vi "Write resource name.vi"(8 "error in (no error)":errorcluster, 10 "resource name":string, 11 "_cameraBase in":refnum<class "_cameraBase.lvclass">) -> (0 "error out":errorcluster, 3 "_cameraBase out":refnum<class "_cameraBase.lvclass">)   [LabVIEW 2018, in "_cameraBase.lvclass"]
uses:
  _cameraBase.lvclass
  _cameraBase.lvclass/_cameraBase.ctl
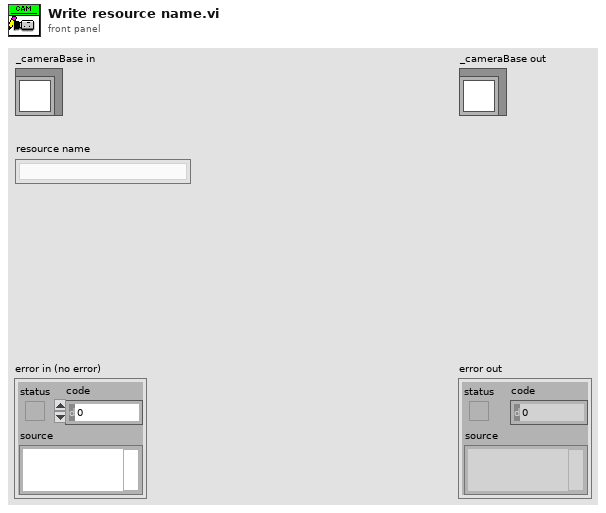
[diagram p1: front panel]
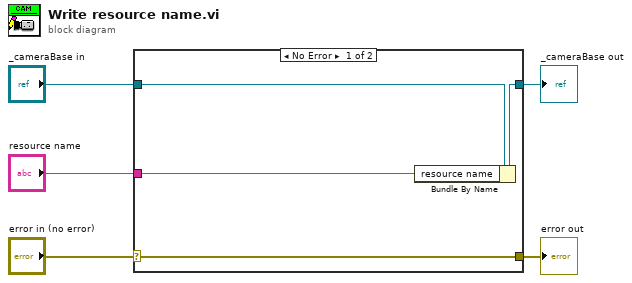
[diagram p0: block diagram]
diagram:
  n1 = case shown="No Error" "error in (no error)" {
    selector: "error in (no error)" -> [w9 w10]
    tunnel: [w9 w10] -> w4
    tunnel: [w7 w11] -> w2
    tunnel: "_cameraBase in" -> [w8 w11]
    tunnel: "resource name" -> [w6 _]
    frame No Error {
      n2 = Bundle By Name(cluster=w8, "resource name"=w6) -> (w7:refnum<class "_cameraBase.lvclass">)
    }
    frame Error {
    }
  }
  "error out" <- w4
  "_cameraBase out" <- w2
